vi "TC Create Task.vi"(8 "error in":errorcluster, 11 "config":T1={"AO config"=[], "AI config"=[], "DI config"=[], "DO config"=[], "TC config"=[], "ACC config"=[], "SG config"=[], "Strain Gauge Settings"={"poisson ratio"=0.3, "nominal gage resistance"=120.0, "gage factor"=2.08}, "bridge information"={"strain configuration"=10271, "lead wire resistance"=1.7, "initial bridge voltage"=0.0, "voltage excitation source"=10200, "voltage excitation value"=3.3}, "Sample Rate"={"AI Sample Rate"=0.0, "AO Sample Rate"=0.0, "DI Sample Rate"=0.0, "TC Sample Rate"=0.0, "DO Sample Rate"=0.0, "SG Sample Rate"=0.0, "ACC Sample Rate"=0.0}} {"bridge information"."initial bridge voltage" format="%0.2f"; "bridge information"."voltage excitation source" items=["Internal"=10200, "External"=10167, "None"=10230]; "bridge information"."voltage excitation value" format="%0.2f"; "bridge information"."lead wire resistance" format="%0.2f"; "bridge information"."strain configuration" items=["Full Bridge I"=10183, "Full Bridge II"=10184, "Full Bridge III"=10185, "Half Bridge I"=10188, "Half Bridge II"=10189, "Quarter Bridge I"=10271, "Quarter Bridge II"=10272]; "ACC config"."Terminal configuration" items=["default"=-1, "RSE"=10083, "NRSE"=10078, "Differential"=10106, "Pseudodifferential"=12529]; "ACC config"."Sensitivity units" items=["mVolts/g"=12509, "Volts/g"=12510]; "TC config"."type" items=["J"=10072, "K"=10073, "N"=10077, "R"=10082, "S"=10085, "T"=10086, "B"=10047, "E"=10055]; "TC config"."units" items=["Deg C", "Deg F", "Kelvins", "Deg R", "From Custom Scale"]}) -> (0 "error out":errorcluster, 2 "empty?":bool, 3 "task out":refnum<k21>)   [LabVIEW 2022 SP3]
uses:
  Controls/Config.ctl
  <vilib>/DAQmx/create/channels.llb/DAQmx Create Channel (AI-Temperature-Thermocouple).vi
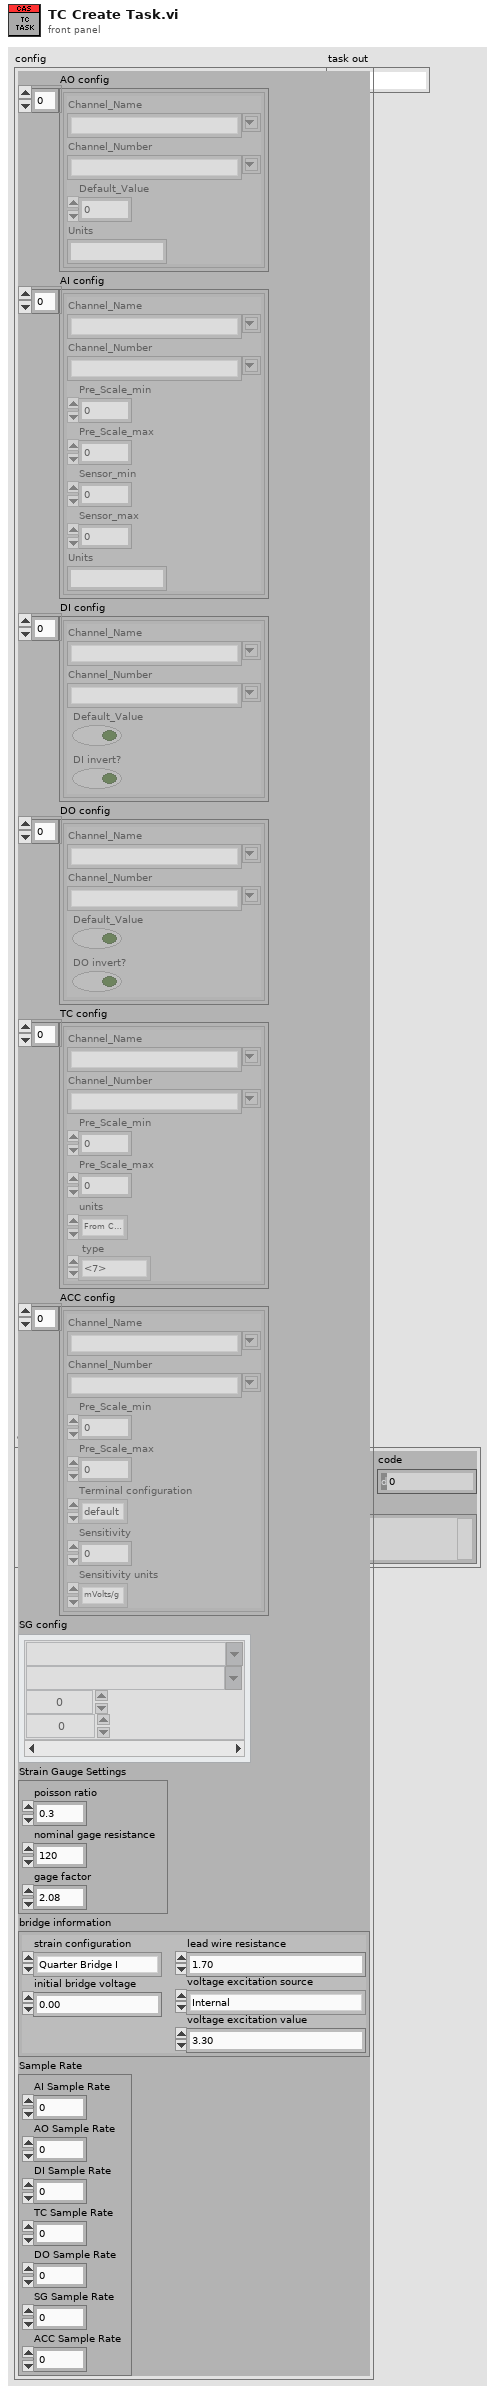
[diagram p1: front panel]
types:
  T1 = typedef "Config.ctl" = cluster{"AO config":cluster{"Channel_Name":string, "Channel_Number":string, "Default_Value":dbl, "Units":string}[], "AI config":cluster{"Channel_Name":string, "Channel_Number":string, "Pre_Scale_min":dbl, "Pre_Scale_max":dbl, "Sensor_min":dbl, "Sensor_max":dbl, "Units":string}[], "DI config":cluster{"Channel_Name":string, "Channel_Number":string, "Default_Value":bool, "DI invert?":bool}[], "DO config":cluster{"Channel_Name":string, "Channel_Number":string, "Default_Value":bool, "DO invert?":bool}[], "TC config":cluster{"Channel_Name":string, "Channel_Number":string, "Pre_Scale_min":dbl, "Pre_Scale_max":dbl, "units":i32, " type":i32}[], "ACC config":cluster{"Channel_Name":string, "Channel_Number":string, "Pre_Scale_min":dbl, "Pre_Scale_max":dbl, "Terminal configuration":i32, "Sensitivity":dbl, "Sensitivity units":i32}[], "SG config":cluster{"Channel_Name":string, "Channel_Number":string, "Pre_Scale_min":dbl, "Pre_Scale_max":dbl}[], "Strain Gauge Settings":cluster{"poisson ratio":dbl, "nominal gage resistance":dbl, "gage factor":dbl}, "bridge information":cluster{"strain configuration":i32, "lead wire resistance":dbl, "initial bridge voltage":dbl, "voltage excitation source":i32, "voltage excitation value":dbl}, "Sample Rate":cluster{"AI Sample Rate":dbl, "AO Sample Rate":dbl, "DI Sample Rate":dbl, "TC Sample Rate":dbl, "DO Sample Rate":dbl, "SG Sample Rate":dbl, "ACC Sample Rate":dbl}}
  T2 = cluster{"Channel_Name":string, "Channel_Number":string, "Pre_Scale_min":dbl, "Pre_Scale_max":dbl, "units":i32, " type":i32}[]
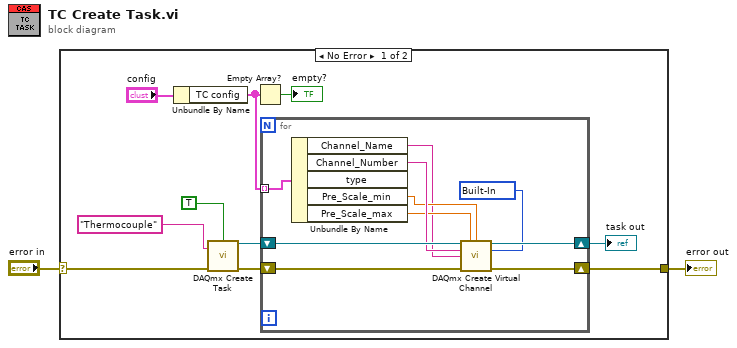
[diagram p0: block diagram]
diagram:
  n1 = case shown="No Error" "error in" {
    selector: "error in" -> [w10 w23]
    tunnel: [w8 w23] -> w1
    frame No Error {
      n2 = Unbundle By Name("config") -> ("TC config"=w6:T2)
      n3 = call <vilib>:"DAQmx Create Task.vi"("new task name"="Thermocouple", "auto cleanup"=TRUE, "error in"=w10) -> ("task out"=w11:refnum<k21>, "error out"=w12:errorcluster)  [unwired: 11 in]
      n4 = Empty Array?(array=w6) -> (empty?=→"empty?":bool)
      n5 = for {
        tunnel: w6 -> [w22] mode=indexing
        shift-right: [w20] -> w9
        shift-left: w11 -> [w21]
        shift-right: [w19] -> w8
        shift-left: w12 -> [w14]
        w13 = 10200 items=["Built-In"=10200, "Constant Value"=10116, "Channel"=10113] ("cjc source")
        n6 = Unbundle By Name(w22) -> ("Channel_Name"=w15:string, "Channel_Number"=w18:string, "Pre_Scale_min"=w16:dbl, "Pre_Scale_max"=w17:dbl)  [unwired: 1 out]
        n7 = call-poly <vilib>:"DAQmx Create Virtual Channel.vi"("task in"=w21, "maximum value"=w17, "minimum value"=w16, "physical channels"=w18, "cjc source"=w13, "name to assign"=w15, "error in"=w14) -> ("task out"=w20:refnum<k21>, "error out"=w19:errorcluster)  [unwired: 7 in]
      }
      "task out" <- w9
    }
    frame Error {
    }
  }
  "error out" <- w1
